vi "Untitled 9 (SubVI).vi"(11 "Array":bool[](array[boolean])) -> (3 "Numeric":i16)   [LabVIEW 2017]
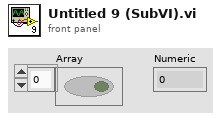
[diagram p1: front panel]
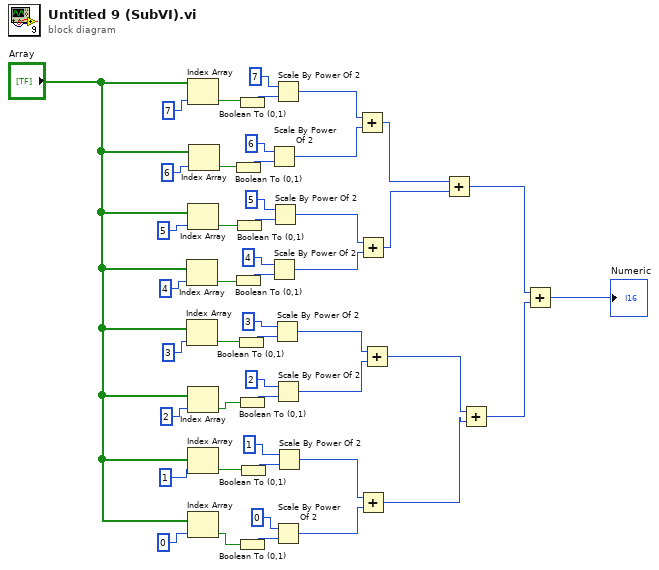
[diagram p0: block diagram]
diagram:
  n1 = Index Array(array="Array", index=4) -> (element=w43:bool)
  n2 = Index Array(array="Array", index=3) -> (element=w32:bool)
  n3 = Index Array(array="Array", index=7) -> (element=w40:bool)
  n4 = Index Array(array="Array", index=5) -> (element=w42:bool)
  n5 = Index Array(array="Array", index=2) -> (element=w44:bool)
  n6 = Index Array(array="Array", index=1) -> (element=w45:bool)
  n7 = Index Array(array="Array", index=0) -> (element=w46:bool)
  n8 = Index Array(array="Array", index=6) -> (element=w41:bool)
  n9 = Boolean To (0,1)(Boolean=w41) -> (0, 1=w7:i16)
  n10 = Boolean To (0,1)(Boolean=w43) -> (0, 1=w5:i16)
  n11 = Boolean To (0,1)(Boolean=w42) -> (0, 1=w6:i16)
  n12 = Boolean To (0,1)(Boolean=w32) -> (0, 1=w4:i16)
  n13 = Boolean To (0,1)(Boolean=w40) -> (0, 1=w8:i16)
  n14 = Boolean To (0,1)(Boolean=w44) -> (0, 1=w3:i16)
  n15 = Boolean To (0,1)(Boolean=w46) -> (0, 1=w1:i16)
  n16 = Boolean To (0,1)(Boolean=w45) -> (0, 1=w2:i16)
  n17 = Scale By Power Of 2(n=6, x=w7) -> (x*2^n=w18:i16)
  n18 = Scale By Power Of 2(n=4, x=w5) -> (x*2^n=w20:i16)
  n19 = Scale By Power Of 2(n=5, x=w6) -> (x*2^n=w19:i16)
  n20 = Scale By Power Of 2(n=3, x=w4) -> (x*2^n=w21:i16)
  n21 = Scale By Power Of 2(n=7, x=w8) -> (x*2^n=w17:i16)
  n22 = Scale By Power Of 2(n=2, x=w3) -> (x*2^n=w22:i16)
  n23 = Scale By Power Of 2(n=0, x=w1) -> (x*2^n=w24:i16)
  n24 = Scale By Power Of 2(n=1, x=w2) -> (x*2^n=w23:i16)
  n25 = Add(x=w17, y=w18) -> (x+y=w28:i16)
  n26 = Add(x=w19, y=w20) -> (x+y=w27:i16)
  n27 = Add(x=w23, y=w24) -> (x+y=w26:i16)
  n28 = Add(x=w21, y=w22) -> (x+y=w25:i16)
  n29 = Add(x=w28, y=w27) -> (x+y=w29:i16)
  n30 = Add(x=w25, y=w26) -> (x+y=w30:i16)
  n31 = Add(x=w29, y=w30) -> (x+y=→"Numeric":i16)
